vi "Condition Name VI.vi"(8 "error in":errorcluster, 9 "Control FP Order":i32[](array[numeric]), 10 "Ref.Name VI":refnum<vi>) -> (0 "error out":errorcluster)   [LabVIEW 2020, in "_Msg Rescript.lvlib" / "_Msg Rescript.lvclass"]
uses:
  _Msg Rescript.lvclass
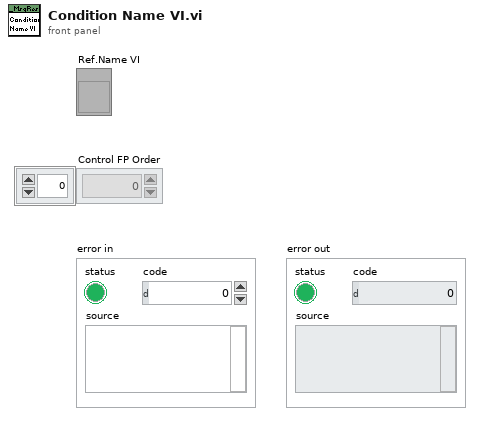
[diagram p1: front panel]
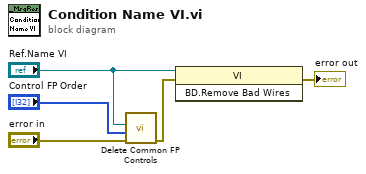
[diagram p0: block diagram]
diagram:
  n1 = call "Delete Common FP Controls.vi"("error in"="error in", "Control FP Order"="Control FP Order", "Ref. VI"="Ref.Name VI") -> ("error out"=w2:errorcluster)  [unwired: 8 in]
  n2 = invoke class="VI" method="BD.Remove Bad Wires"(reference="Ref.Name VI", error in=w2) -> (error out=→"error out":errorcluster)  [unwired: 1 in, 2 out]
